vi "Render Axes.vi"(8 "error in (no error)":errorcluster, 11 "Main Controller Actor in":refnum<class "Main Controller Actor.lvclass">) -> (0 "error out":errorcluster)   [LabVIEW 2021, in "Main Controller Actor.lvclass"]
uses:
  Main Controller Actor.lvclass
  Main Controller Actor.lvclass/Main Controller Actor.ctl
  LabSDL2/Source/Libraries/LibSDL2 Wrapper/LibSDL2.lvlib
  LabSDL2/Source/Libraries/SDL2 Utility/Point (I32).ctl
  LabSDL2/Source/Libraries/SDL2 Utility/SDL2 Utility.lvlib
  Camera/Camera.lvclass
  Vector 2D/Vector 2D.lvclass
  Renderer/Renderer.lvclass
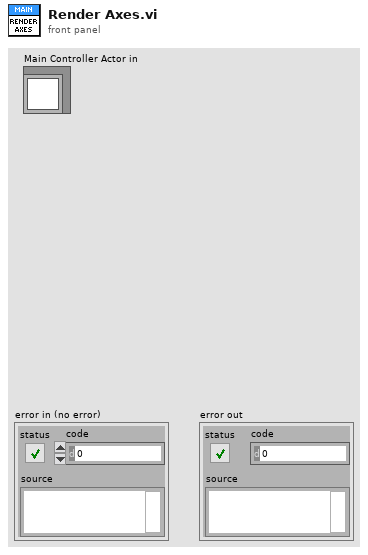
[diagram p1: front panel]
types:
  T1 = typedef "SDL2 Utility.lvlib/Point (I32).ctl" = cluster{"x":i32, "y":i32}
  T2 = typedef "Constants.ctl" = cluster{"Colours":cluster{"OK":u32, "Warning":u32, "Error":u32, "Red":u32, "Green":u32, "Blue":u32, "Yellow":u32}, "System":cluster{"Target Frames Second":dbl, "World Size":T1, "Window Size":T1, "Battle Area Size":T1, "Sidebar Scaling":sgl, "Sidebar Width":i32, "SC2 Frame Rate [Seconds/Frame]":sgl}, "Game":cluster{"Maximum Asteroids":i32, "Max Energy":i32, "Max Crew":i32, "Maximum Stars":i32}}
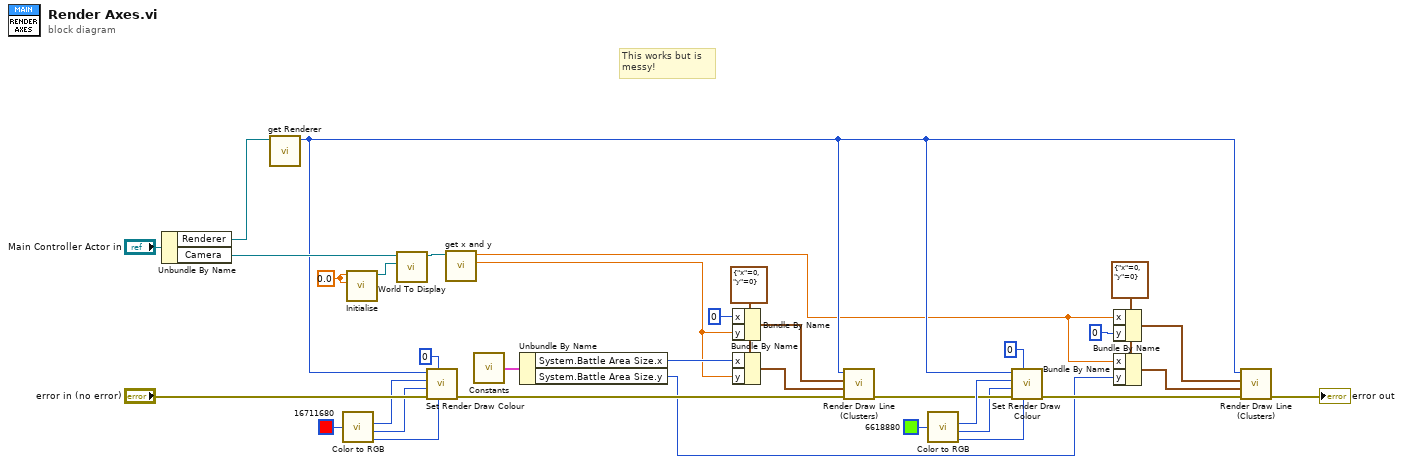
[diagram p0: block diagram]
diagram:
  w5 = sgl 0.0 ("x")
  w21 = T1 {"x"=0, "y"=0} ("Start")
  w27 = T1 {"x"=0, "y"=0} ("Start")
  # "This works but is messy!"
  n1 = Unbundle By Name("Main Controller Actor in") -> ("Renderer"=w6:refnum<class "Renderer.lvclass">, "Camera"=w8:refnum<class "Camera.lvclass">)
  n2 = call-dynamic "get Renderer.vi"("Renderer in"=w6) -> ("Renderer"=w7:u32)  [unwired: 10 in]
  n3 = call <vilib>:"Color to RGB.vi"("Color"=u32 16711680) -> ("R"=w33:u8, "G"=w32:u8, "B"=w31:u8)  [unwired: 1 out]
  n4 = call "Initialise.vi"("y"=w5, "x"=w5) -> ("Vector 2D out"=w4:refnum<class "Vector 2D.lvclass">)  [unwired: 9 in]
  n5 = call "World To Display.vi"("World Position"=w4, "Camera in"=w8) -> ("Display Position"=w3:refnum<class "Vector 2D.lvclass">)  [unwired: 9 in]
  n6 = call "Set Render Draw Colour.vi"("B"=w31, "A"=u8 0, "error in (no error)"="error in (no error)", "G"=w32, "R"=w33, "Renderer Pointer"=w7) -> ("error out"=w30:errorcluster)  [unwired: 4 in, 1 out]
  n7 = call "get x and y.vi"("Vector 2D in"=w3) -> ("y"=w1:sgl, "x"=w2:sgl)  [unwired: 9 in]
  n8 = call "Constants.vi"() -> ("Constants"=w11:T2)
  n9 = Unbundle By Name(w11) -> ("System.Battle Area Size.x"=w10:i32, "System.Battle Area Size.y"=w9:i32)
  n10 = Bundle By Name(cluster=w27, "x"=0 ("y"), "y"=w1) -> (w26:T1)
  n11 = Bundle By Name(cluster=w27, "x"=w10, "y"=w1) -> (w25:T1)
  n12 = call "Render Draw Line (Clusters).vi"("error in"=w30, "End"=w25, "Start"=w26, "Renderer Pointer"=w7) -> ("error out"=w15:errorcluster)  [unwired: 6 in, 1 out]
  n13 = call <vilib>:"Color to RGB.vi"("Color"=u32 6618880) -> ("R"=w17:u8, "G"=w13:u8, "B"=w12:u8)  [unwired: 1 out]
  n14 = call "Set Render Draw Colour.vi"("B"=w12, "A"=u8 0, "error in (no error)"=w15, "G"=w13, "R"=w17, "Renderer Pointer"=w7) -> ("error out"=w14:errorcluster)  [unwired: 4 in, 1 out]
  n15 = Bundle By Name(cluster=w21, "x"=w2, "y"=0) -> (w22:T1)
  n16 = Bundle By Name(cluster=w21, "x"=w2, "y"=w9) -> (w23:T1)
  n17 = call "Render Draw Line (Clusters).vi"("error in"=w14, "End"=w23, "Start"=w22, "Renderer Pointer"=w7) -> ("error out"=→"error out":errorcluster)  [unwired: 6 in, 1 out]
